vi "Manual Scale.vi"(8 "error in (no error)":errorcluster, 9 "Secs/div":dbl, 10 "V/div":T1, 11 "PXIe5105 in":refnum<class "PXIe5105.lvclass">) -> (0 "error out":errorcluster, 3 "PXIe5105 out":refnum<class "PXIe5105.lvclass">)   [LabVIEW 2018, in "PXIe5105.lvlib" / "PXIe5105.lvclass"]
doc: "This Overrride is used to manually adjust the scale of the instrument."
uses:
  PXIe5105.lvclass
  PPLs/Oscilloscope/Parent/Oscilloscope.lvlibp/Custom Controls/Volts per Division.ctl
  PPLs/Oscilloscope/Parent/Oscilloscope.lvlibp/Custom Controls/Analog Channels.ctl
  PPLs/Oscilloscope/Parent/Oscilloscope.lvlibp
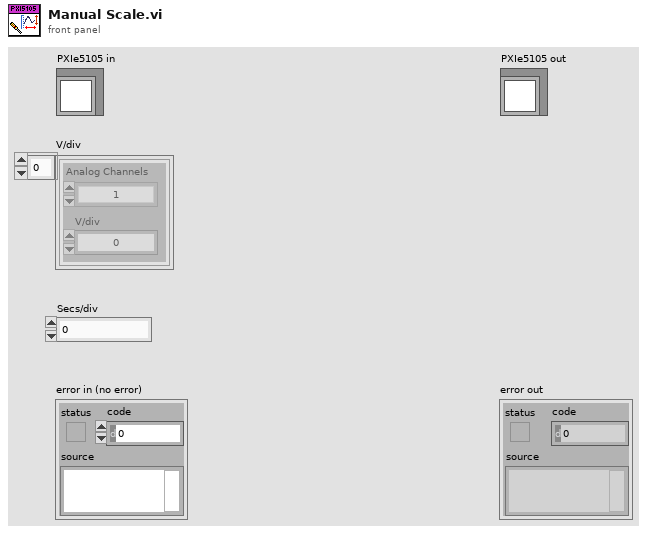
[diagram p1: front panel]
types:
  T1 = typedef "Oscilloscope.lvlibp/Volts per Division.ctl" = cluster{"Analog Channels":T2, "V/div":dbl}[]
  T2 = typedef "Oscilloscope.lvlibp/Analog Channels.ctl" = enum16{"1", "2", "3", "4", "5", "6", "7", "8", "9", "10", "11", "12", "13", "14", "15", "16"}
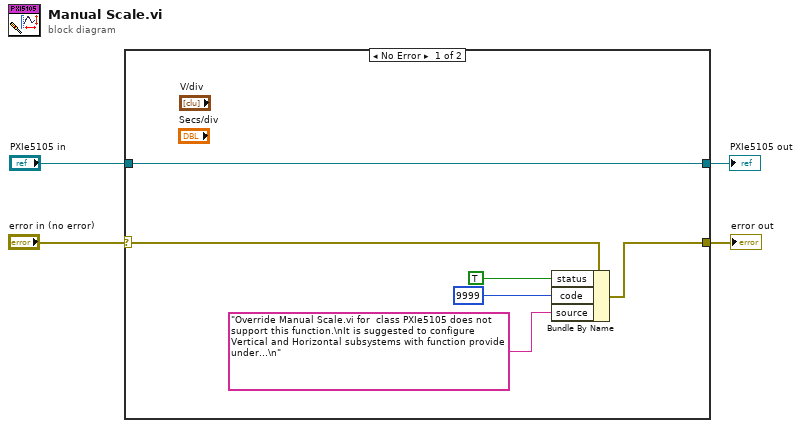
[diagram p0: block diagram]
diagram:
  n1 = case shown="No Error" "error in (no error)" {
    selector: "error in (no error)" -> [w6 w12]
    tunnel: [w5 w12] -> w3
    tunnel: [w10 w11] -> w2
    tunnel: "PXIe5105 in" -> [w10 w11]
    frame No Error {
      n2 = Bundle By Name(cluster=w6, "status"=TRUE, "code"=9999, "source"="Override Manual Scale.vi for  class PXIe5105 does not support this function.\nIt is suggested to configure Vertical and Horizontal subsystems with function provide under...\n") -> (w5:errorcluster)
    }
    frame Error {
    }
  }
  "error out" <- w3
  "PXIe5105 out" <- w2
